vi "ProcessingJournalEvent.vi"(8 "error IO":errorcluster, 9 "Новая строка в журнале":string, 10 "Журнал событий":refnum<vi>, 11 "ArchiveInput":refnum<class "Archive.lvclass">) -> (3 "Archive Out":refnum<class "Archive.lvclass">)   [LabVIEW 2010]
uses:
  Archive.lvclass
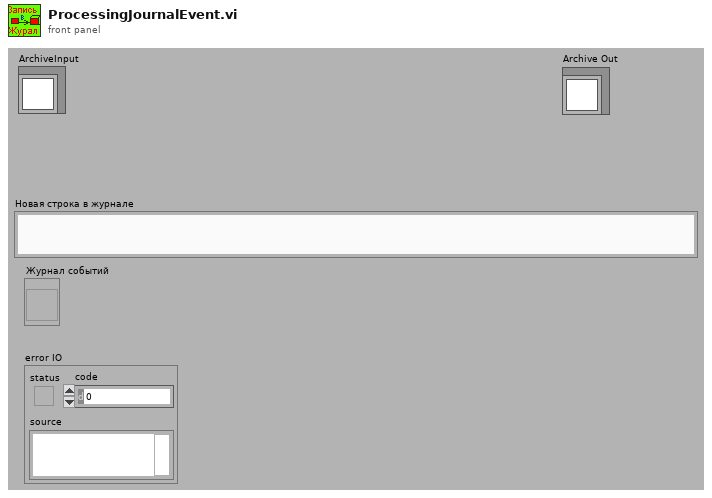
[diagram p1: front panel]
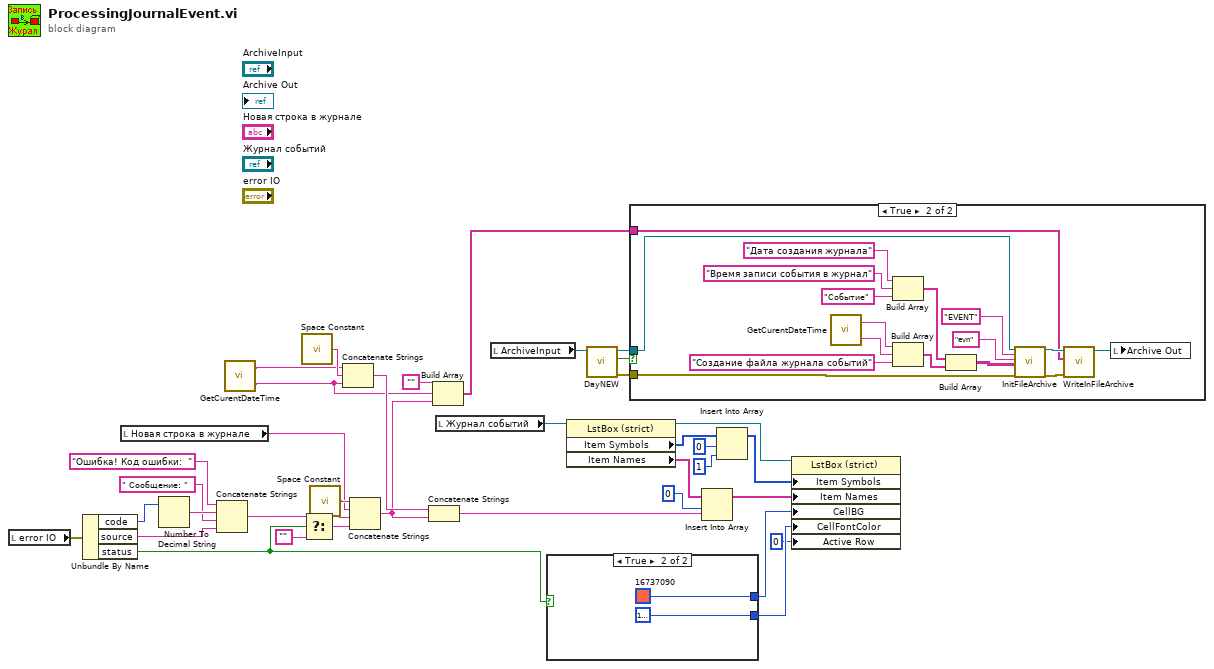
[diagram p0: block diagram]
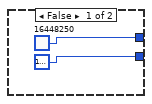
[diagram p2: hidden frame]
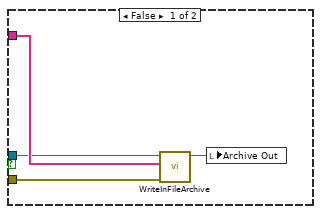
[diagram p3: hidden frame]
diagram:
  n1 = local read "error IO"() -> (w32:errorcluster)
  n2 = Unbundle By Name(w32) -> ("code"=w23:i32, "source"=w19:string, "status"=w4:bool)
  n3 = local read "Новая строка в журнале"() -> (w12:string)
  n4 = Number To Decimal String(number=w23) -> (decimal integer string=w21:string)  [unwired: 1 in]
  n5 = Concatenate Strings("Ошибка! Код ошибки:  " ("t"), w21, " Сообщение: " ("t"), w19) -> (w18:string)
  n6 = call "GetCurentDateTime.vi"() -> ("time"=w5:string, "date"=w6:string)  [unwired: 2 in]
  n7 = call <vilib>:"Space Constant.vi"() -> ("String"=w16:string)
  n8 = Select(t=w18, s=w4, f="") -> (s? t:f=w31:string)
  n9 = call <vilib>:"Space Constant.vi"() -> ("String"=w30:string)
  n10 = Concatenate Strings(w6, w16, w5) -> (w14:string)
  n11 = Concatenate Strings(w30, w12, w30, w31) -> (w13:string)
  n12 = Concatenate Strings(w14, w13) -> (w15:string)
  n13 = Build Array("", w5, w13) -> (w8:string[])
  n14 = local read "Журнал событий"() -> (w35:refnum<vi>)
  n15 = local read "ArchiveInput"() -> (w11:refnum<class "Archive.lvclass">)
  n16 = case shown="True" w4 {
    tunnel: [u32 16448250 u32 16737090] -> w3
    tunnel: [u32 16777222 u32 16777222] -> w2
    frame False {
    }
    frame True {
    }
  }
  n17 = property class="LstBox (strict)"(reference=w35) -> (reference out=w34:refnum<vi>, "Item Symbols"=w29:i32[], "Item Names"=w28:string[])  [unwired: 1 in, 1 out]
  n18 = call-dynamic "DayNEW.vi"("Archive in"=w11) -> ("error out"=w7:errorcluster, "NewDay"=w10:bool, "Archive out"=w9:refnum<class "Archive.lvclass">)  [unwired: 8 in]
  n19 = case shown="True" w10 {
    tunnel: w9 -> [w41 w52]
    tunnel: w8 -> [w44 w49]
    tunnel: w7 -> [w43 w47]
    frame False {
      n20 = call-dynamic "WriteInFileArchive.vi"("error in (no error)"=w43, "Строка таблицы"=w44, "Archive in"=w41) -> ("Archive out"=w42:refnum<class "Archive.lvclass">)  [unwired: 7 in, 1 out]
      n21 = local write "Archive Out"(w42) -> ()
    }
    frame True {
      n22 = call "GetCurentDateTime.vi"() -> ("time"=w45:string, "date"=w46:string)  [unwired: 2 in]
      n23 = Build Array("Дата создания журнала", "Время записи события в журнал", "Событие" ("element")) -> (w58:string[])
      n24 = Build Array(w46, w45, "Создание файла журнала событий" ("element")) -> (w54:string[])
      n25 = Build Array(w58, w54) -> (w61:string[][])
      n26 = call-dynamic "InitFileArchive.vi"("Archive In"=w52, "Имя папки"="EVENT", "Расширение имени файла"="evn", "Заголовок таблицы"=w61, "error in (no error)"=w47) -> ("Archive out"=w51:refnum<class "Archive.lvclass">, "error out"=w50:errorcluster)  [unwired: 13 in]
      n27 = call-dynamic "WriteInFileArchive.vi"("error in (no error)"=w50, "Строка таблицы"=w49, "Archive in"=w51) -> ("Archive out"=w48:refnum<class "Archive.lvclass">)  [unwired: 7 in, 1 out]
      n28 = local write "Archive Out"(w48) -> ()
    }
  }
  n29 = Insert Into Array(array=w28, index=0, new element=w15) -> (w26:string[])
  n30 = Insert Into Array(array=w29, index=0, new element=1 ("new element/subarray")) -> (w27:i32[])
  n31 = property class="LstBox (strict)"(reference=w34, "Item Symbols"=w27, "Item Names"=w26, "CellBG"=w3, "CellFontColor"=w2, "Active Row"=0 ("Active Row:Active Row Number")) -> ()  [unwired: 1 in, 2 out]
